vi "VMExport.vi"(8 "error in (no error)":errorcluster, 11 "VariableManagerRef in":refnum<vi>) -> (0 "error out":errorcluster, 2 "VariableManagerExportCopy":refnum<class "VariableManager.lvclass">, 3 "VariableManagerRef out":refnum<vi>)   [LabVIEW 2013, in "VariableManagerAPI.lvlib"]
doc: "Export a copy of VariableManager object from the reference.\nAny change on this object will not affect the object of the reference."
uses:
  VariableManagerAPI.lvlib
  VariableManager/VariableManager.lvclass
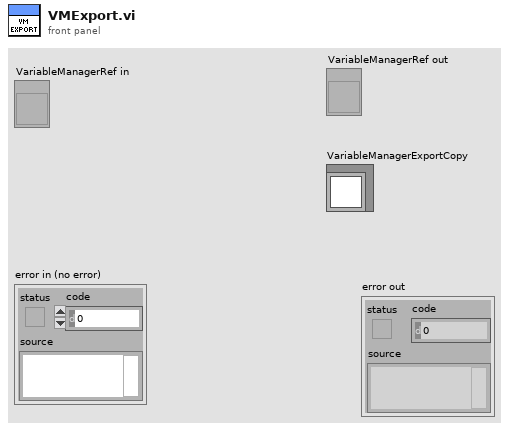
[diagram p1: front panel]
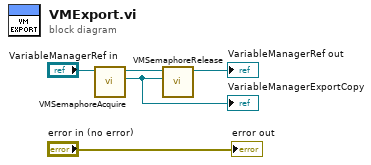
[diagram p0: block diagram]
diagram:
  n1 = call "VMSemaphoreAcquire.vi"("VariableManagerRef in"="VariableManagerRef in") -> ("VariableManager"=w1:refnum<class "VariableManager.lvclass">, "VariableManagerRef out"=w3:refnum<vi>)  [unwired: 7 in, 2 out]
  "VariableManagerExportCopy" <- w1
  n2 = call "VMSemaphoreRelease.vi"("VariableManager"=w1, "VariableManagerRef in"=w3) -> ("VariableManagerRef out"=→"VariableManagerRef out":refnum<vi>)  [unwired: 8 in, 1 out]
  "error out" <- "error in (no error)"
